vi "KeyboardControl.vi"(8 "Array":i32[](array[numeric])=[0, 0], 9 "NxN":i32, 10 "which action":i32, 11 "Initial arraIy":picture[][](array[picture])) -> (1 "result mark blank":i32[](array[numeric]), 2 "Result array 2":picture[][](array[picture]))   [LabVIEW 2014]
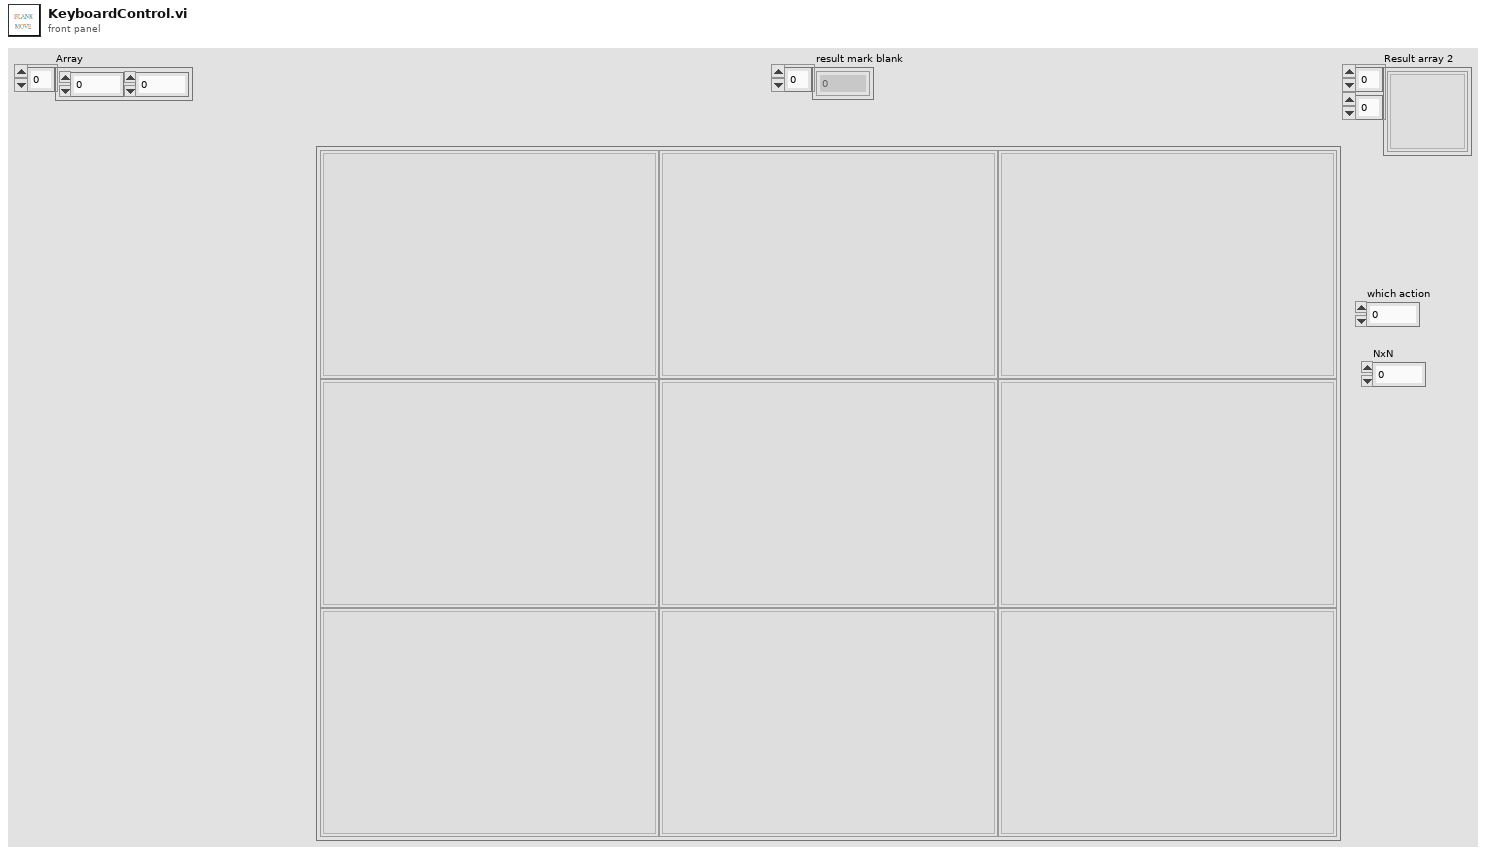
[diagram p1: front panel]
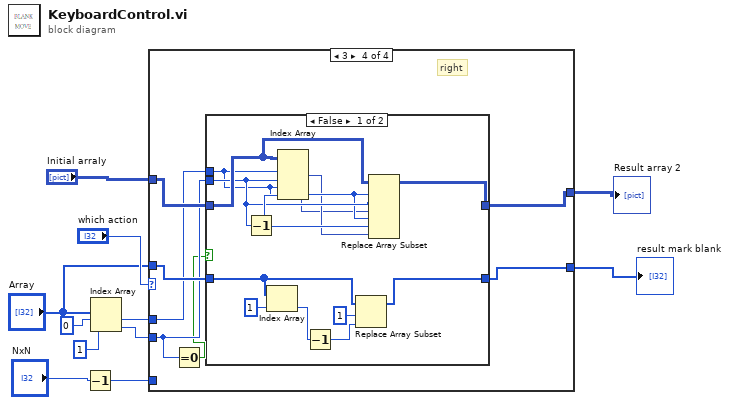
[diagram p0: block diagram]
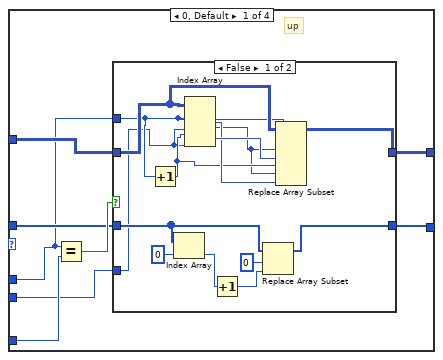
[diagram p2: hidden frame]
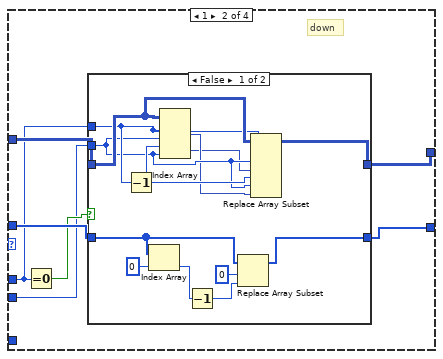
[diagram p4: hidden frame]
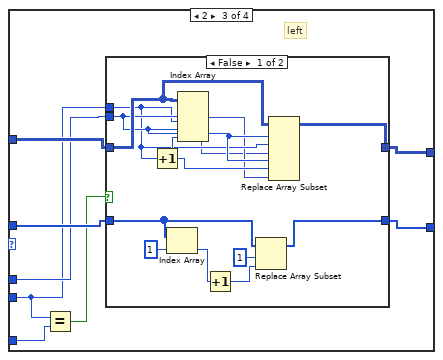
[diagram p6: hidden frame]
diagram:
  n1 = Decrement(x="NxN") -> (x-1=w7:i32)
  n2 = Index Array(array="Array", index #1=0 ("index"), index #2=1 ("index")) -> (element #1=w6:i32, element #2=w1:i32)
  n3 = case shown="3" "which action" {
    tunnel: w7 -> [w13 _ w58 _]
    tunnel: w6 -> [w14 w36 w60 w84]
    tunnel: [w18 w38 w61 w83] -> w4
    tunnel: "Array" -> [w17 w40 w63 w85]
    tunnel: "Initial arraIy" -> [w16 w41 w64 w86]
    tunnel: [w15 w39 w62 w82] -> w2
    tunnel: w1 -> [w12 w35 w59 w81]
    frame 0, Default {
      # "up"
      n4 = Equal?(x=w14, y=w13) -> (x = y?=w19:bool)
      n5 = case shown="False" w19 {
        tunnel: [w29 w34] -> w18
        tunnel: w17 -> [w30 w34]
        tunnel: w16 -> [w32 w33]
        tunnel: [w31 w33] -> w15
        tunnel: w14 -> [w24 _]
        tunnel: w12 -> [w20 _]
        frame False {
          n6 = Increment(x=w24) -> (x+1=w21:i32)
          n7 = Index Array(array=w30, index=0) -> (element=w25:i32)
          n8 = Index Array(array=w32, index (row) #1=w24, index (col) #1=w20, index (row) #2=w21, index (col) #2=w20) -> (element #1=w22:picture, element #2=w23:picture)
          n9 = Increment(x=w25) -> (x+1=w26:i32)
          n10 = Replace Array Subset(array=w30, new element=w26, index=0) -> (w29:i32[])
          n11 = Replace Array Subset(array=w32, new element #1=w23, index (row) #1=w24, index (col) #1=w20, new element #2=w22, index (row) #2=w21, index (col) #2=w20) -> (w31:picture[][])
        }
        frame True {
        }
      }
    }
    frame 1 {
      # "down"
      n12 = Equal To 0?(x=w36) -> (x = 0?=w37:bool)
      n13 = case shown="False" w37 {
        tunnel: [w51 w56] -> w38
        tunnel: w40 -> [w52 w56]
        tunnel: w41 -> [w54 w55]
        tunnel: [w53 w55] -> w39
        tunnel: w36 -> [w46 _]
        tunnel: w35 -> [w44 _]
        frame False {
          n14 = Decrement(x=w46) -> (x-1=w45:i32)
          n15 = Index Array(array=w52, index=0) -> (element=w47:i32)
          n16 = Index Array(array=w54, index (row) #1=w46, index (col) #1=w44, index (row) #2=w45, index (col) #2=w44) -> (element #1=w43:picture, element #2=w42:picture)
          n17 = Decrement(x=w47) -> (x-1=w48:i32)
          n18 = Replace Array Subset(array=w52, new element=w48, index=0) -> (w51:i32[])
          n19 = Replace Array Subset(array=w54, new element #1=w42, index (row) #1=w46, index (col) #1=w44, new element #2=w43, index (row) #2=w45, index (col) #2=w44) -> (w53:picture[][])
        }
        frame True {
        }
      }
    }
    frame 2 {
      # "left"
      n20 = Equal?(x=w59, y=w58) -> (x = y?=w57:bool)
      n21 = case shown="False" w57 {
        tunnel: [w74 w79] -> w61
        tunnel: w63 -> [w75 w79]
        tunnel: w64 -> [w77 w78]
        tunnel: [w76 w78] -> w62
        tunnel: w60 -> [w69 _]
        tunnel: w59 -> [w67 _]
        frame False {
          n22 = Increment(x=w67) -> (x+1=w68:i32)
          n23 = Index Array(array=w75, index=1) -> (element=w70:i32)
          n24 = Index Array(array=w77, index (row) #1=w69, index (col) #1=w67, index (row) #2=w69, index (col) #2=w68) -> (element #1=w66:picture, element #2=w65:picture)
          n25 = Increment(x=w70) -> (x+1=w71:i32)
          n26 = Replace Array Subset(array=w75, new element=w71, index=1) -> (w74:i32[])
          n27 = Replace Array Subset(array=w77, new element #1=w65, index (row) #1=w69, index (col) #1=w67, new element #2=w66, index (row) #2=w69, index (col) #2=w68) -> (w76:picture[][])
        }
        frame True {
        }
      }
    }
    frame 3 {
      # "right"
      n28 = Equal To 0?(x=w81) -> (x = 0?=w80:bool)
      n29 = case shown="False" w80 {
        tunnel: [w96 w101] -> w83
        tunnel: w85 -> [w97 w101]
        tunnel: w86 -> [w99 w100]
        tunnel: [w98 w100] -> w82
        tunnel: w84 -> [w89 _]
        tunnel: w81 -> [w90 _]
        frame False {
          n30 = Decrement(x=w90) -> (x-1=w91:i32)
          n31 = Index Array(array=w97, index=1) -> (element=w92:i32)
          n32 = Index Array(array=w99, index (row) #1=w89, index (col) #1=w90, index (row) #2=w89, index (col) #2=w91) -> (element #1=w88:picture, element #2=w87:picture)
          n33 = Decrement(x=w92) -> (x-1=w93:i32)
          n34 = Replace Array Subset(array=w97, new element=w93, index=1) -> (w96:i32[])
          n35 = Replace Array Subset(array=w99, new element #1=w87, index (row) #1=w89, index (col) #1=w90, new element #2=w88, index (row) #2=w89, index (col) #2=w91) -> (w98:picture[][])
        }
        frame True {
        }
      }
    }
  }
  "result mark blank" <- w4
  "Result array 2" <- w2
